vi "BuildSelectQuery.vi"(8 "error in (no error)":errorcluster, 10 "QueryBuilderData":T1) -> (0 "error out":errorcluster, 2 "Query":string)   [LabVIEW 2022 SP3]
uses:
  DataTypes/QuiryBuilderData--Cluster.ctl
  <vilib>/Utility/error.llb/Trim Whitespace One-Sided.vi
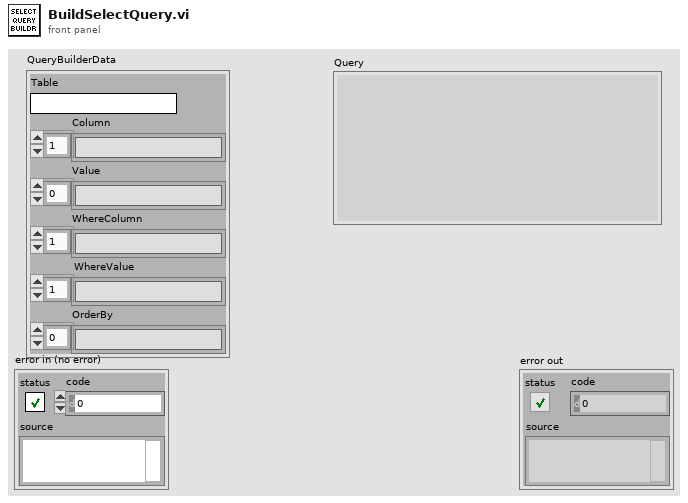
[diagram p1: front panel]
types:
  T1 = typedef "QuiryBuilderData--Cluster.ctl" = cluster{"Table":string, "Column":string[], "Value":string[], "WhereColumn":string[], "WhereValue":string[], "OrderBy":string[]}
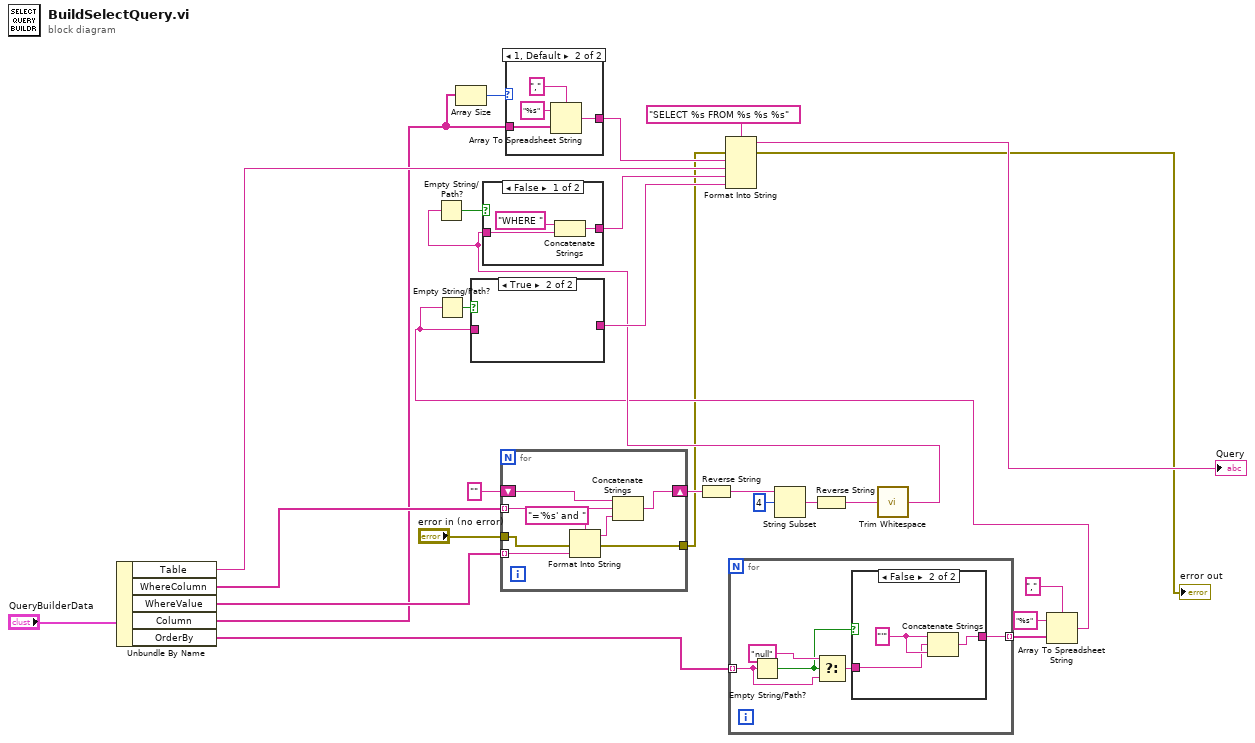
[diagram p0: block diagram]
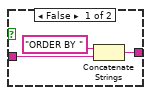
[diagram p2: hidden frame]
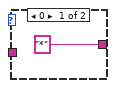
[diagram p4: hidden frame]
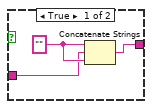
[diagram p5: hidden frame]
diagram:
  n1 = Unbundle By Name("QueryBuilderData") -> ("Table"=w7:string, "WhereColumn"=w16:string[], "WhereValue"=w17:string[], "Column"=w6:string[], "OrderBy"=w5:string[])
  n2 = Array Size(array=w6) -> (size(s)=w14:i32)
  n3 = for {
    tunnel: w16 -> [w36] mode=indexing
    shift-right: [w35] -> w24
    shift-left: "" -> [w34]
    tunnel: w17 -> [w31] mode=indexing
    tunnel: "error in (no error)" -> [w30]
    tunnel: [w29] -> w1
    n4 = Format Into String(format string="='%s' and " ("string"), error in=w30, w31) -> (resulting string=w32:string, error out=w29:errorcluster)  [unwired: 1 in]
    n5 = Concatenate Strings(w34, w36, w32) -> (w35:string)
  }
  n6 = case shown="1, Default" w14 {
    tunnel: ["*" ("CommandText") w38] -> w13
    tunnel: w6 -> [_ w41]
    frame 0 {
    }
    frame 1, Default {
      n7 = Array To Spreadsheet String(delimiter (Tab)=",", array=w41, 3:"%s" ("format string")) -> (spreadsheet string=w38:string)
    }
  }
  n8 = Reverse String(1:w24) -> (0:w22:string)
  n9 = for {
    tunnel: w5 -> [w43] mode=indexing
    tunnel: [w46] -> w28 mode=indexing
    n10 = Empty String/Path?(string/path=w43) -> (empty?=w42:bool)
    n11 = Select(t="null" ("string"), s=w42, f=w43) -> (s? t:f=w45:string)
    n12 = case shown="False" w42 {
      tunnel: [w48 w51] -> w46
      tunnel: w45 -> [w47 w50]
      frame True {
        w49 = "" ("string")
        n13 = Concatenate Strings(w49, w47, w49) -> (w48:string)
      }
      frame False {
        w52 = "'" ("string")
        n14 = Concatenate Strings(w52, w50, w52) -> (w51:string)
      }
    }
  }
  n15 = String Subset(string=w22, offset (0)=4) -> (substring=w21:string)  [unwired: 1 in]
  n16 = Reverse String(1:w21) -> (0:w20:string)
  n17 = call <vilib>:"Trim Whitespace.vi"("string"=w20) -> ("trimmed string"=w8:string)  [unwired: 1 in]
  n18 = Empty String/Path?(string/path=w8) -> (empty?=w12:bool)
  n19 = case shown="False" w12 {
    tunnel: w8 -> [w55 _]
    tunnel: [w53 _] -> w11
    frame False {
      n20 = Concatenate Strings("WHERE " ("string"), w55) -> (w53:string)
    }
    frame True {
    }
  }
  n21 = Array To Spreadsheet String(delimiter (Tab)=",", array=w28, 3:"%s" ("format string")) -> (spreadsheet string=w4:string)
  n22 = Empty String/Path?(string/path=w4) -> (empty?=w10:bool)
  n23 = case shown="True" w10 {
    tunnel: w4 -> [w58 _]
    tunnel: [w56 _] -> w9
    frame False {
      n24 = Concatenate Strings("ORDER BY " ("string"), w58) -> (w56:string)
    }
    frame True {
    }
  }
  n25 = Format Into String(format string="SELECT %s FROM %s %s %s" ("CommandText"), error in=w1, w13, w7, w11, w9) -> (resulting string=→"Query":string, error out=→"error out":errorcluster)  [unwired: 1 in]
